vi "Variant_UpdateElements.vi"(10 "New Element(s)":variant, 11 "Original Element(s)":variant) -> (3 "Merged Elements":variant)   [LabVIEW 2013, in "OpenVariant.lvlib"]
uses:
  OpenVariant.lvlib
  TypeDescriptor/TypeDescriptor_GetPString.vi
  TypeDescriptor/OpenDescriptor.lvlib
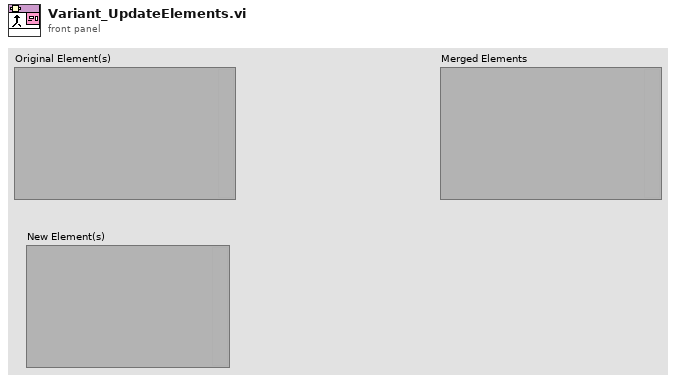
[diagram p1: front panel]
types:
  T1 = typedef "OpenDescriptor.lvlib/Descriptor Element -- cluster.ctl" = cluster{"type descriptor":i16[], "name":string, "class":string, "data string":string}
  T2 = typedef "Type Descriptor I16 Array.ctl" = T3[]
  T3 = typedef "Type Descriptor I16.ctl" = i16
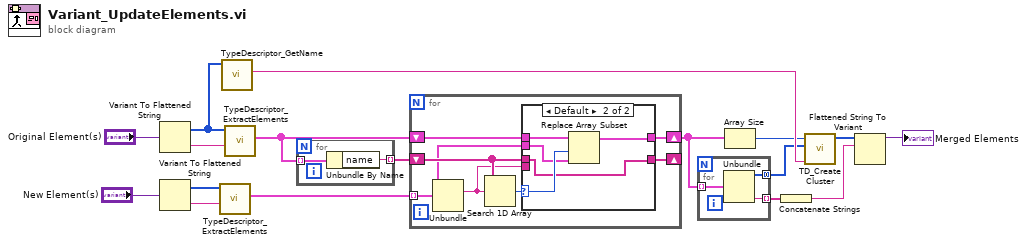
[diagram p0: block diagram]
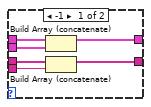
[diagram p2: hidden frame]
diagram:
  n1 = Variant To Flattened String(Variant="Original Element(s)") -> (data string=w4:string, 1:w16:i16[])
  n2 = Variant To Flattened String(Variant="New Element(s)") -> (data string=w1:string, 1:w14:i16[])
  n3 = call "TypeDescriptor_ExtractElements.vi"("Data String"=w1, "type descriptor"=w14) -> ("elements"=w10:T1[])  [unwired: 6 in, 3 out]
  n4 = call "TypeDescriptor_GetName.vi"("type descriptor"=w16) -> ("name"=w11:string)  [unwired: 8 in, 2 out]
  n5 = call "TypeDescriptor_ExtractElements.vi"("Data String"=w4, "type descriptor"=w16) -> ("elements"=w9:T1[])  [unwired: 6 in, 3 out]
  n6 = for {
    tunnel: w9 -> [w19] mode=indexing
    tunnel: [w18] -> w8 mode=indexing
    n7 = Unbundle By Name(w19) -> ("name"=w18:string)
  }
  n8 = for {
    tunnel: w10 -> [w20] mode=indexing
    shift-right: [w25] -> w6
    shift-left: w9 -> [w26]
    shift-right: [w22] -> _
    shift-left: w8 -> [w24]
    n9 = Unbundle(w20) -> ("name"=w23:string)  [unwired: 3 out]
    n10 = Search 1D Array(1D array=w24, element=w23) -> (index of element=w21:i32)  [unwired: 1 in]
    n11 = case shown="Default" w21 {
      selector: w21 -> [_ w36]
      tunnel: w26 -> [w32 w37]
      tunnel: w20 -> [w31 w35]
      tunnel: [w30 w34] -> w25
      tunnel: w24 -> [w29 w33]
      tunnel: w23 -> [w28 _]
      tunnel: [w27 w33] -> w22
      frame -1 {
        n12 = Build Array (concatenate)(w32, w31) -> (w30:T1[])
        n13 = Build Array (concatenate)(w29, w28) -> (w27:string[])
      }
      frame Default {
        n14 = Replace Array Subset(array=w37, new element=w35, index=w36) -> (w34:T1[])
      }
    }
  }
  n15 = for {
    tunnel: w6 -> [w40] mode=indexing
    tunnel: [w39] -> w7 mode=concatenating
    tunnel: [w38] -> w3 mode=indexing
    n16 = Unbundle(w40) -> ("type descriptor"=w39:i16[], "data string"=w38:string)  [unwired: 2 out]
  }
  n17 = Array Size(array=w6) -> (size(s)=w5:i32)
  n18 = Concatenate Strings(w3) -> (w2:string)
  n19 = call <vilib>:"TD_Create Cluster.vi"("Name"=w11, "Concatenated Elts"=w7, "N Elts"=w5) -> ("ClusterTD"=w17:T2)  [unwired: 8 in]
  n20 = Flattened String To Variant(6:w2, 7:w17) -> (3:→"Merged Elements":variant)  [unwired: 1 in, 1 out]
